vi "lockinOptimiser.vi"() -> ()   [LabVIEW 2014]
uses:
  <vilib>/Utility/file.llb/Read From Spreadsheet File (DBL).vi
  <userlib>/Nanonis Prog Interface V5/Nanonis Prog Interface.lvlib
  <vilib>/Analysis/NI_AALBase.lvlib
  <vilib>/gmath/NI_Gmath.lvlib
panel:
  in  "Number of points":i32=250
  in  "End Frequency (Hz)":dbl=250.0
  in  "Start Frequency (Hz)":dbl=250.0
  in  "Direction to flow through array":enum16{"Normal", "Reverse", "Random"}(ring)
  out "Std Dev":cluster{"all rows":dbl[], dbl[]}[](graph)
  out "SNR":cluster{"all rows":dbl[], dbl[]}[](graph)
  out "all rows":dbl[][](array[numeric]) format="%0.3f"
  out "Demod":cluster{"all rows":dbl[], dbl[]}[](graph)
  in  "Settling Time (s)":dbl=1000.0
  in  "Integration Time (s)":dbl=600.0
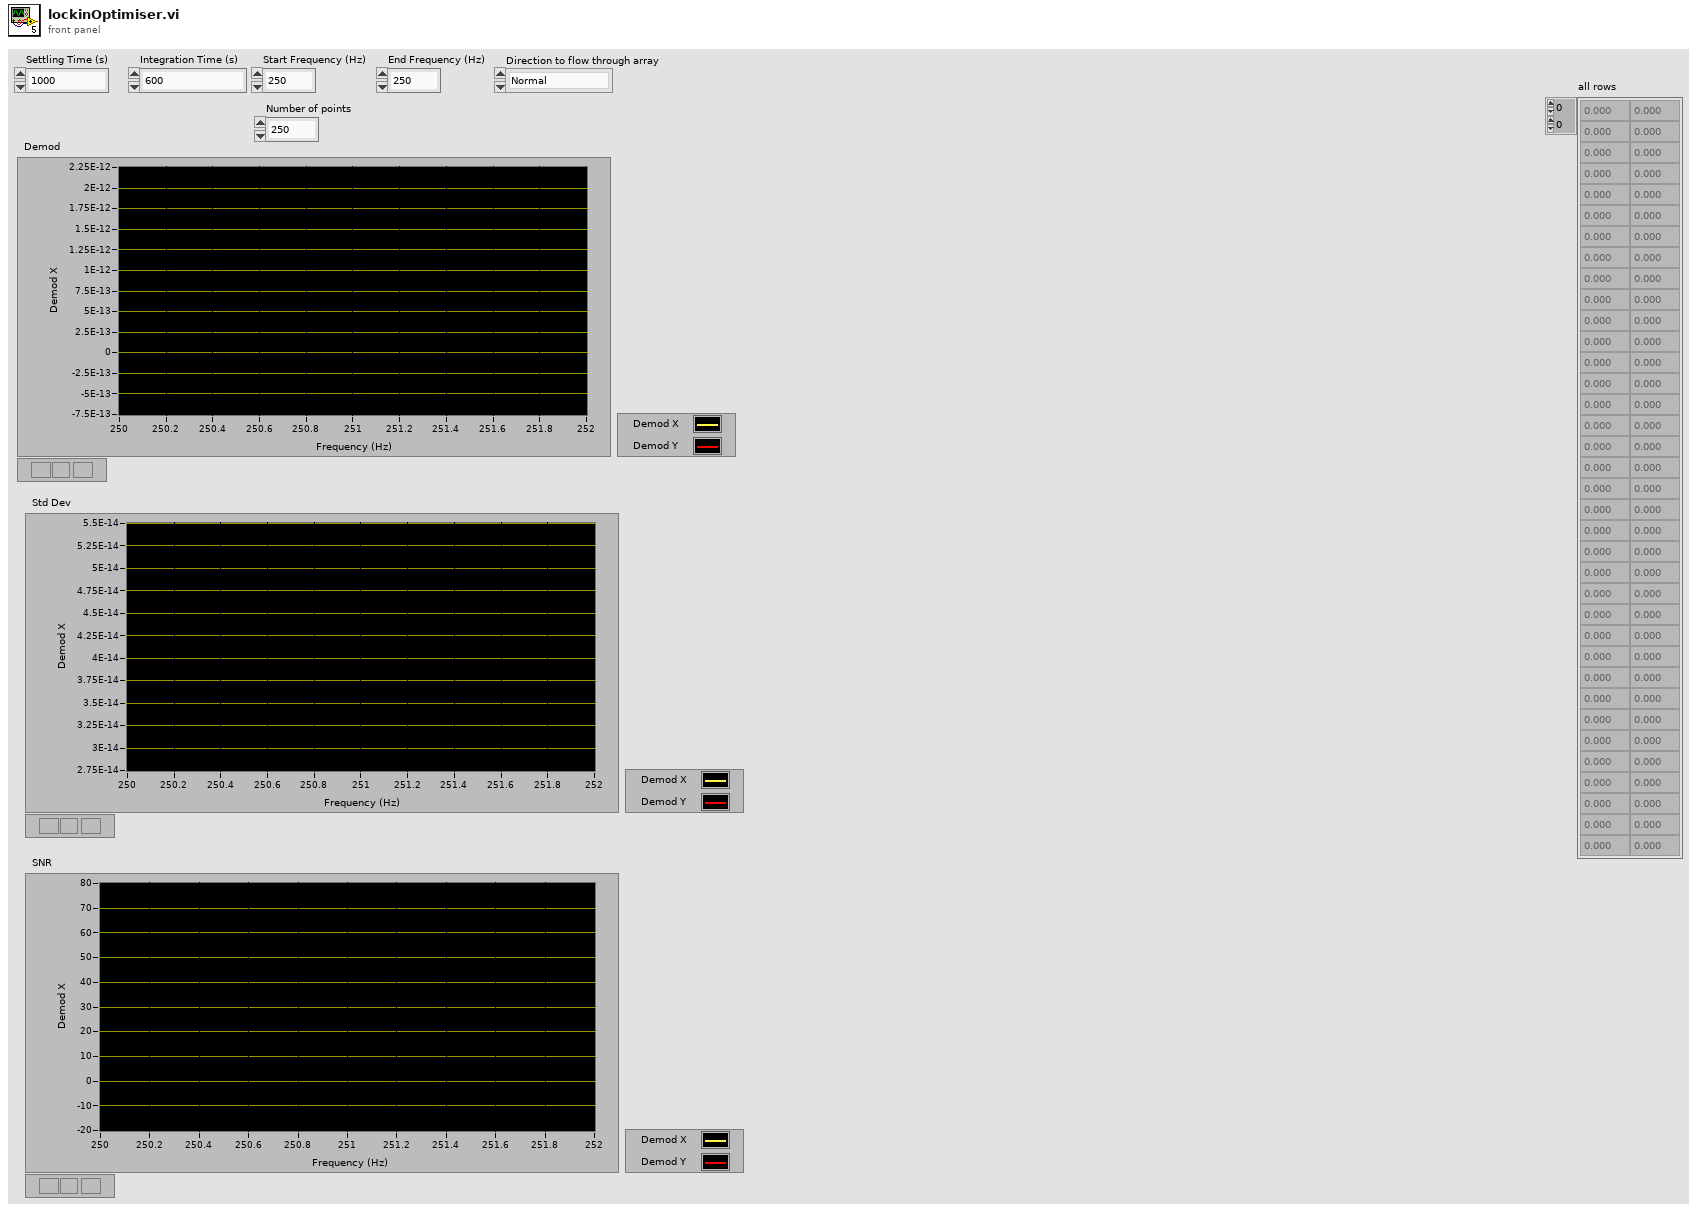
[diagram p1: front panel]
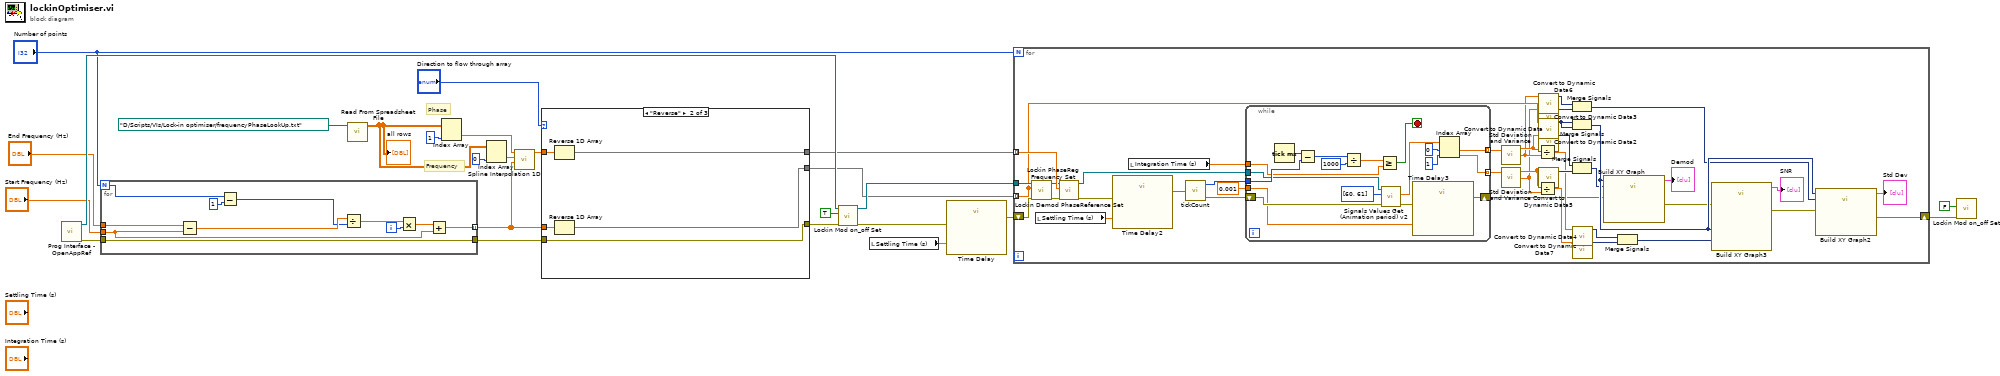
[diagram p0: block diagram]
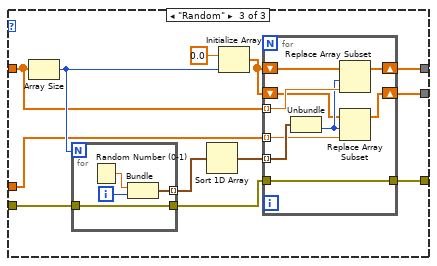
[diagram p3: hidden frame]
diagram:
  # "Frequency"
  # "Phase"
  n1 = call <userlib>:"Prog Interface - OpenAppRef.vi"() -> ("Error out"=w3:errorcluster, "Application reference"=w21:refnum<vi>)  [unwired: 6 in]
  n2 = for {
    N: "Number of points" -> [w34]
    tunnel: "End Frequency (Hz)" -> [w36]
    tunnel: "Start Frequency (Hz)" -> [w28]
    tunnel: [w27] -> w5 mode=indexing
    tunnel: [w26] -> w2
    tunnel: w3 -> [w26]
    i -> [w30]
    n3 = Subtract(x=w36, y=w28) -> (x-y=w35:dbl)
    n4 = Subtract(x=w34, y=1) -> (x-y=w32:i32)
    n5 = Divide(x=w35, y=w32) -> (x/y=w31:dbl)
    n6 = Multiply(x=w31, y=w30) -> (x*y=w29:dbl)
    n7 = Add(x=w29, y=w28) -> (x+y=w27:dbl)
  }
  n8 = call-poly <vilib>:"Read From Spreadsheet File.vi"("file path (dialog if empty)"=path "D:/Scripts/VIs/Lock-in optimiser/frequencyPhaseLookUp.txt") -> ("all rows"=w20:dbl[][])  [unwired: 6 in, 4 out]
  "all rows" <- w20
  n9 = Index Array(array=w20, index (col)=1 ("index")) -> (element=w7:dbl[])  [unwired: 1 in]
  n10 = Index Array(array=w20, index (col)=0 ("index")) -> (element=w8:dbl[])  [unwired: 1 in]
  n11 = call <vilib>:"Spline Interpolation 1D.vi"("xi"=w5, "X"=w8, "Y"=w7) -> ("yi"=w6:dbl[])  [unwired: 6 in, 2 out]
  n12 = case shown="\"Reverse\"" "Direction to flow through array" {
    tunnel: w6 -> [w39 w44 w52]
    tunnel: [w39 w43 w49] -> w12
    tunnel: w5 -> [w38 w42 w51]
    tunnel: [w38 w41 w50] -> w11
    tunnel: w2 -> [w37 w40 w47]
    tunnel: [w37 w40 w45] -> w1
    frame "Normal", Default {
    }
    frame "Reverse" {
      n13 = Reverse 1D Array(array=w44) -> (reversed array=w43:dbl[])
      n14 = Reverse 1D Array(array=w42) -> (reversed array=w41:dbl[])
    }
    frame "Random" {
      n15 = Array Size(array=w52) -> (size(s)=w53:i32)
      n16 = for {
        N: w53 -> [_]
        tunnel: [w59] -> w54 mode=indexing
        tunnel: w47 -> [w57]
        tunnel: [w57] -> w46
        i -> [w60]
        n17 = Random Number (0-1)() -> (number: 0 to 1=w58:dbl)
        n18 = Bundle("number: 0 to 1"=w58, w60) -> (w59:cluster{"number: 0 to 1":dbl, i32})  [unwired: 1 in]
      }
      n19 = Sort 1D Array(array=w54) -> (sorted array=w55:cluster{"number: 0 to 1":dbl, i32}[])
      n20 = Initialize Array(0.0 ("element"), w53) -> (w48:dbl[])
      n21 = for {
        tunnel: w55 -> [w69] mode=indexing
        shift-right: [w68] -> w49
        shift-left: w48 -> [w65]
        tunnel: w52 -> [w67] mode=indexing
        tunnel: w51 -> [w66] mode=indexing
        shift-right: [w63] -> w50
        shift-left: w48 -> [w62]
        tunnel: w46 -> [w61]
        tunnel: [w61] -> w45
        n22 = Unbundle(w69) -> (w64:i32)  [unwired: 1 out]
        n23 = Replace Array Subset(array=w65, new element=w67, index=w64) -> (w68:dbl[])
        n24 = Replace Array Subset(array=w62, new element=w66, index=w64) -> (w63:dbl[])
      }
    }
  }
  n25 = call <userlib>:"Lockin Mod on_off Set.vi"("Error in (no error)"=w1, "Lockin ON/OFF"=TRUE, "Application ref in"=w21) -> ("Error out"=w16:errorcluster, "Application ref out"=w22:refnum<vi>)  [unwired: 7 in]
  n26 = local read "Settling Time (s)"() -> (w15:dbl)
  n27 = call "Time Delay"("error in (no error)"=w16, "Delay Time (s)"=w15) -> ("error out"=w14:errorcluster)  [unwired: 9 in]
  n28 = for {
    N: "Number of points" -> [_]
    tunnel: w11 -> [w97] mode=indexing
    tunnel: w12 -> [w109] mode=indexing
    tunnel: w22 -> [w108]
    shift-right: [w75] -> w24
    shift-left: w14 -> [w106]
    n29 = call <userlib>:"Lockin PhaseReg Frequency Set.vi"("Error in (no error)"=w106, "Frequency (Hz)"=w97, "Application ref in"=w108) -> ("Error out"=w105:errorcluster, "Application ref out"=w107:refnum<vi>)  [unwired: 7 in]
    n30 = local read "Settling Time (s)"() -> (w73:dbl)
    n31 = call <userlib>:"Lockin Demod PhaseReference Set.vi"("Error in (no error)"=w105, "Phase Reference"=w109, "Application ref in"=w107) -> ("Error out"=w74:errorcluster, "Application ref out"=w102:refnum<vi>)  [unwired: 7 in]
    n32 = call "Time Delay2"("error in (no error)"=w74, "Delay Time (s)"=w73) -> ("error out"=w71:errorcluster)  [unwired: 9 in]
    n33 = local read "Integration Time (s)"() -> (w103:dbl)
    n34 = call "tickCount.vi"("error in (no error)"=w71) -> ("error out"=w70:errorcluster, "millisecond timer value"=w72:u32)
    n35 = while {
      tunnel: w72 -> [w127]
      tunnel: 0.001 ("Integration Time (ms)") -> [w113]
      tunnel: w103 -> [w124]
      tunnel: w102 -> [w123]
      tunnel: [w117] -> w101 mode=indexing
      tunnel: [w116] -> w100 mode=indexing
      shift-right: [w114] -> w78
      shift-left: w70 -> [w122]
      stop <- w125 stop-if-true
      n36 = Tick Count (ms)() -> (millisecond timer value=w126:u32)
      n37 = Subtract(x=w126, y=w127) -> (x-y=w112:u32)
      n38 = Divide(x=w112, y=u32 1000) -> (x/y=w111:dbl)
      n39 = Greater Or Equal?(x=w111, y=w124) -> (x >= y?=w125:bool)
      n40 = call <userlib>:"Signals Values Get (Animation period) v2.vi"("error in (no error)"=w122, "Signals indexes (0-79)"=i8[] [60, 61], "Application ref in"=w123) -> ("error out"=w115:errorcluster, "Signals Values"=w120:sgl[])  [unwired: 5 in, 1 out]
      n41 = call "Time Delay3"("error in (no error)"=w115, "Delay Time (s)"=w113) -> ("error out"=w114:errorcluster)  [unwired: 9 in]
      n42 = Index Array(array=w120, index #1=0 ("index"), index #2=1 ("index")) -> (element #1=w117:sgl, element #2=w116:sgl)
    }
    n43 = call <vilib>:"Std Deviation and Variance.vi"("X"=w101) -> ("mean"=w85:dbl, "standard deviation"=w84:dbl)  [unwired: 1 in, 1 out]
    n44 = call <vilib>:"Std Deviation and Variance.vi"("X"=w100) -> ("mean"=w83:dbl, "standard deviation"=w82:dbl)  [unwired: 1 in, 1 out]
    n45 = Divide(x=w85, y=w84) -> (x/y=w86:dbl)
    n46 = Divide(x=w83, y=w82) -> (x/y=w81:dbl)
    n47 = call "Convert to Dynamic Data6"("Double"=w84) -> ("Dynamic Data Type"=w92:dynamicdata)  [unwired: 3 in]
    n48 = call "Convert to Dynamic Data3"("Double"=w82) -> ("Dynamic Data Type"=w91:dynamicdata)  [unwired: 3 in]
    n49 = call "Convert to Dynamic Data"("Double"=w97) -> ("Dynamic Data Type"=w99:dynamicdata)  [unwired: 3 in]
    n50 = call "Convert to Dynamic Data2"("Double"=w85) -> ("Dynamic Data Type"=w95:dynamicdata)  [unwired: 3 in]
    n51 = call "Convert to Dynamic Data5"("Double"=w83) -> ("Dynamic Data Type"=w94:dynamicdata)  [unwired: 3 in]
    n52 = Merge Signals(w92, w91) -> (w90:dynamicdata)
    n53 = Merge Signals(w99, w99) -> (w98:dynamicdata)
    n54 = Merge Signals(w95, w94) -> (w93:dynamicdata)
    n55 = call "Convert to Dynamic Data4"("Double"=w86) -> ("Dynamic Data Type"=w89:dynamicdata)  [unwired: 3 in]
    n56 = call "Convert to Dynamic Data7"("Double"=w81) -> ("Dynamic Data Type"=w88:dynamicdata)  [unwired: 3 in]
    n57 = call "Build XY Graph"("error in (no error)"=w78, "Y Input"=w93, "X Input"=w98) -> ("error out"=w77:errorcluster, "XY Graph"=→"Demod":cluster{"X":dbl[], "Y":dbl[]}[])  [unwired: 7 in]
    n58 = Merge Signals(w89, w88) -> (w87:dynamicdata)
    n59 = call "Build XY Graph3"("error in (no error)"=w77, "Y Input"=w87, "X Input"=w98) -> ("error out"=w76:errorcluster, "XY Graph"=→"SNR":cluster{"X":dbl[], "Y":dbl[]}[])  [unwired: 7 in]
    n60 = call "Build XY Graph2"("error in (no error)"=w76, "Y Input"=w90, "X Input"=w98) -> ("error out"=w75:errorcluster, "XY Graph"=→"Std Dev":cluster{"X":dbl[], "Y":dbl[]}[])  [unwired: 7 in]
  }
  n61 = call <userlib>:"Lockin Mod on_off Set.vi"("Error in (no error)"=w24, "Lockin ON/OFF"=FALSE) -> ()  [unwired: 8 in, 2 out]
